vi "Read Status Msg.vi"(8 "error in (no error)":errorcluster, 11 "Session Handle in":T1) -> (0 "error out":errorcluster, 2 "Status Msg":string, 3 "Session Handle out":T1)   [LabVIEW 2018, in "Process Bar.lvclass"]
uses:
  Process Bar.lvclass
  Typedefs/Session Handle.ctl
  Process Bar.lvclass/Process Bar.ctl
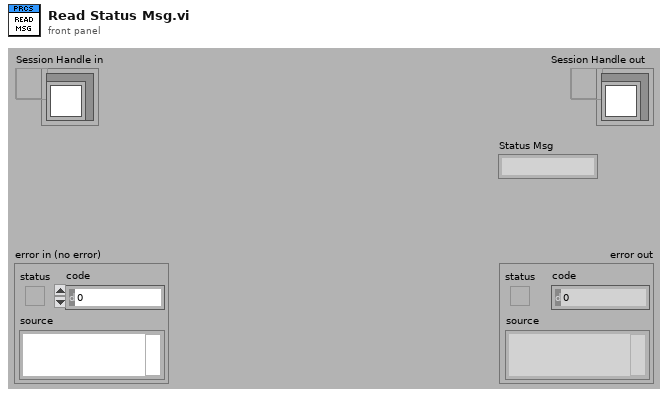
[diagram p1: front panel]
types:
  T1 = typedef "Process Bar.lvclass/Session Handle.ctl" = refnum<data-value>
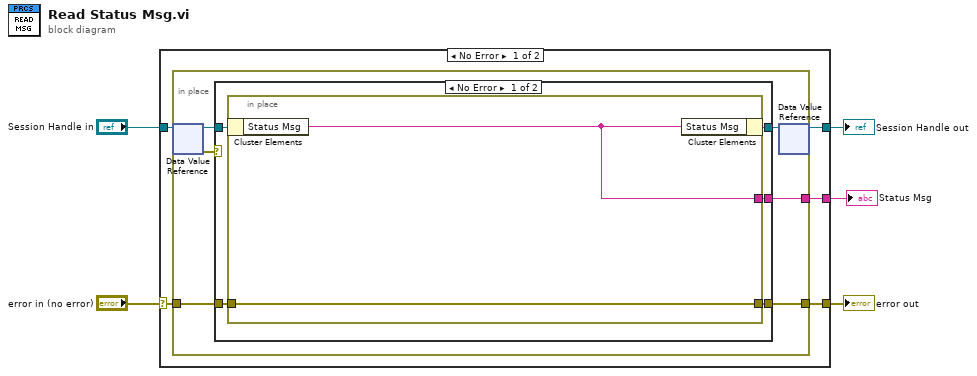
[diagram p0: block diagram]
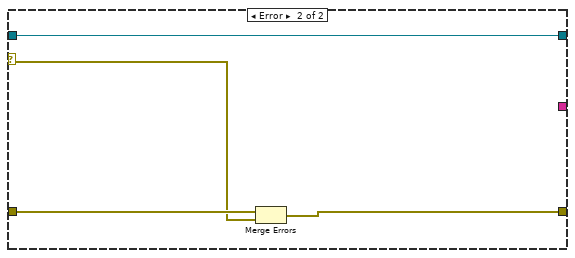
[diagram p2: hidden frame]
diagram:
  n1 = case shown="No Error" "error in (no error)" {
    selector: "error in (no error)" -> [w8 w28]
    tunnel: "Session Handle in" -> [w10 w29]
    tunnel: [w9 w29] -> w4
    tunnel: [w7 w28] -> w3
    tunnel: [w6 _] -> w1
    frame No Error {
      n2 = in-place {
        in-place-border: w8 -> [w12]
        in-place-border: [w15] -> w7
        in-place-border: [w11] -> w6
        n3 = in-place-dvr #1(w10) -> (w16:refnum<class "Process Bar.lvclass">, w13:errorcluster)
        n4 = case shown="No Error" w13 {
          selector: w13 -> [_ w26]
          tunnel: w16 -> [w21 w24]
          tunnel: [w20 w25] -> w15
          tunnel: [w19 w24] -> w14
          tunnel: w12 -> [w18 w27]
          tunnel: [w17 _] -> w11
          frame No Error {
            n5 = in-place {
              in-place-border: [w23] -> w20
              in-place-border: w18 -> [w23]
              in-place-border: [w22] -> w17
              n6 = in-place-cluster #2(w21) -> ("Status Msg"=w22:string)
              n7 = in-place-cluster #2("Status Msg"=w22) -> (w19:refnum<class "Process Bar.lvclass">)
            }
          }
          frame Error {
            n8 = Merge Errors(w27, w26) -> (w25:errorcluster)
          }
        }
        n9 = in-place-dvr #1(w14) -> (w9:T1)  [unwired: 1 out]
      }
    }
    frame Error {
    }
  }
  "Session Handle out" <- w4
  "error out" <- w3
  "Status Msg" <- w1
